vi "Rango_Max_Min.vi"() -> ()   [LabVIEW 2020]
panel:
  out "LED":bool
  out "Arreglo":dbl[](array[numeric])
  out "Valor escalar":dbl
  in  "Min":dbl
  in  "Max":dbl
  # "Diego Jáuregui Ontiveros\nCarlos Uriel Casas Casas\nAlejandro López González"
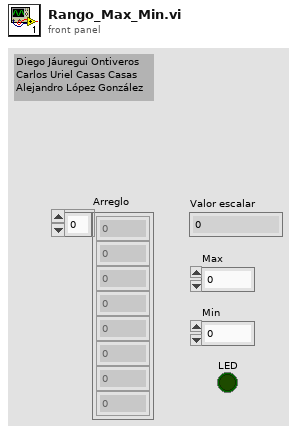
[diagram p1: front panel]
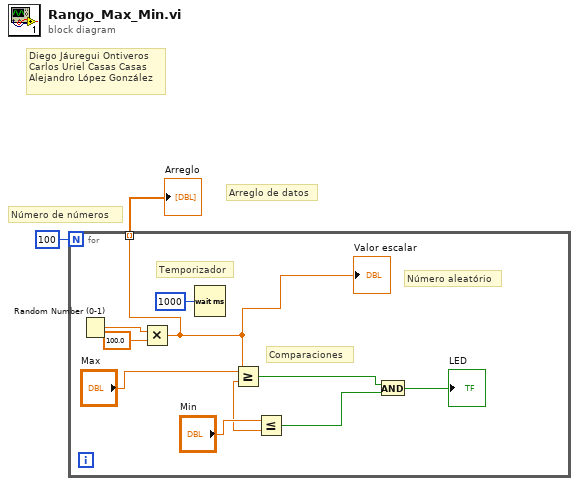
[diagram p0: block diagram]
diagram:
  # "Arreglo de datos"
  # "Número de números"
  # "Diego Jáuregui Ontiveros\nCarlos Uriel Casas Casas\nAlejandro López González"
  n1 = for {
    N: 100 -> [_]
    tunnel: [w4] -> w1 mode=indexing
    # "Comparaciones"
    # "Número aleatório"
    # "Temporizador"
    n2 = Random Number (0-1)() -> (number: 0 to 1=w10:dbl)
    n3 = Multiply(x=w10, y=100.0) -> (x*y=w4:dbl)
    "Valor escalar" <- w4
    n4 = Wait (ms)(milliseconds to wait=u32 1000) -> ()  [unwired: 1 out]
    n5 = Greater Or Equal?(x="Max", y=w4) -> (x >= y?=w6:bool)
    n6 = Less Or Equal?(x="Min", y=w4) -> (x <= y?=w5:bool)
    n7 = And(x=w6, y=w5) -> (x .and. y?=→"LED":bool)
  }
  "Arreglo" <- w1
